vi "Flush Queue.vi"(8 "error in (no error)":errorcluster, 11 "QDMH in":refnum<class "QDMH.lvclass">) -> (0 "error out":errorcluster, 2 "Flushed Elements":T1[](array[typedef]), 3 "QDMH out":refnum<class "QDMH.lvclass">)   [LabVIEW 2023, in "QDMH.lvlib" / "QDMH.lvclass"]
doc: "Flush queue returns all the elements in the queue stack\n\nIt is usefor for processing large quantities of enqueued elements in bulk when dequeing individually is too time intensive for processing."
uses:
  Library/QDMH.lvclass
  Custom Controls/Message.ctl
  Library/QDMH.lvclass/QDMH.ctl
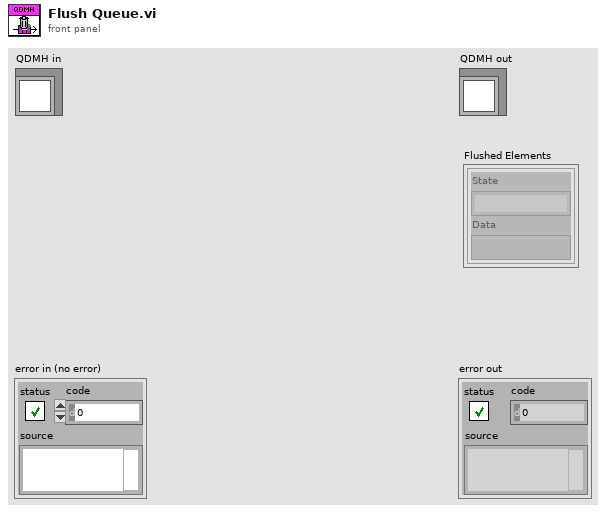
[diagram p1: front panel]
types:
  T1 = typedef "QDMH.lvlib/QDMH.lvclass/Message.ctl" = cluster{"State":string, "Data":variant}
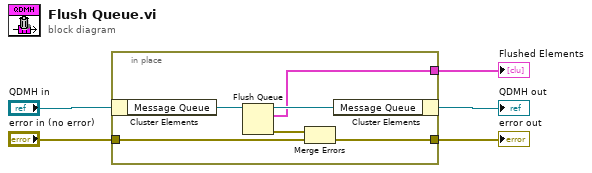
[diagram p0: block diagram]
diagram:
  n1 = in-place {
    in-place-border: "error in (no error)" -> [w8]
    in-place-border: [w7] -> w3
    in-place-border: [w6] -> w1
    n2 = in-place-cluster #1("QDMH in") -> ("Message Queue"=w11:refnum<queue>)
    n3 = Flush Queue(queue=w11) -> (queue out=w10:refnum<queue>, remaining elements=w6:T1[], error out=w9:errorcluster)  [unwired: 1 in]
    n4 = Merge Errors(w9, w8) -> (w7:errorcluster)
    n5 = in-place-cluster #1("Message Queue"=w10) -> (→"QDMH out":refnum<class "QDMH.lvclass">)
  }
  "error out" <- w3
  "Flushed Elements" <- w1
